vi "Autonomous Path Planner.vi"() -> ()   [LabVIEW 2016]
uses:
  <vilib>/Utility/miscctls.llb/LVCursorListTypeDef.ctl
  <vilib>/Analysis/1siggen.llb/Ramp Pattern by Samples.vi
  Common Code/Utilities/Change Detect String.vi
  <vilib>/Analysis/NI_AALBase.lvlib
  <vilib>/Analysis/NI_AALPro.lvlib
panel:
  in  "Field Lines":T1(array[cluster])=[{"X"=-326.0, "Y"=122.875, "X 2"=-322.0, "Y 2"=122.875}, {"X"=-326.0, "Y"=121.125, "X 2"=-322.0, "Y 2"=121.125}, {"X"=-326.0, "Y"=52.125, "X 2"=-322.0, "Y 2"=52.125}, {"X"=-326.0, "Y"=50.375, "X 2"=-322.0, "Y 2"=50.375}, {"X"=-326.0, "Y"=20.375, "X 2"=-322.0, "Y 2"=20.375}, {"X"=-326.0, "Y"=18.625, "X 2"=-322.0, "Y 2"=18.625}, {"X"=-326.0, "Y"=-50.375, "X 2"=-322.0, "Y 2"=-50.375}, {"X"=-326.0, "Y"=-52.125, "X 2"=-322.0, "Y 2"=-52.125}, {"X"=-326.0, "Y"=-121.125, "X 2"=-322.0, "Y 2"=-121.125}, {"X"=-326.0, "Y"=-122.875, "X 2"=-322.0, "Y 2"=-122.875}, {"X"=0.0, "Y"=0.0, "X 2"=0.0, "Y 2"=0.0}, {"X"=-211.7, "Y"=-20.5, "X 2"=-211.7, "Y 2"=20.5}, {"X"=-140.7, "Y"=-20.5, "X 2"=-140.7, "Y 2"=20.5}, {"X"=-176.2, "Y"=41.0, "X 2"=-211.7, "Y 2"=20.5}, {"X"=-176.2, "Y"=41.0, "X 2"=-140.7, "Y 2"=20.5}, {"X"=-176.2, "Y"=-41.0, "X 2"=-211.7, "Y 2"=-20.5}, {"X"=-176.2, "Y"=-41.0, "X 2"=-140.7, "Y 2"=-20.4}, {"X"=-326.0, "Y"=-126.0, "X 2"=-290.0, "Y 2"=-162.0}, {"X"=-326.0, "Y"=126.0, "X 2"=-254.0, "Y 2"=162.0}, {"X"=-247.5, "Y"=-162.0, "X 2"=-247.5, "Y 2"=-158.0}, {"X"=-221.3, "Y"=-162.0, "X 2"=-221.3, "Y 2"=-158.0}, {"X"=-191.3, "Y"=-162.0, "X 2"=-191.3, "Y 2"=-158.0}, {"X"=-165.1, "Y"=-162.0, "X 2"=-165.1, "Y 2"=-158.0}, {"X"=-41.2, "Y"=-162.0, "X 2"=-41.2, "Y 2"=-158.0}, {"X"=-15.0, "Y"=-162.0, "X 2"=-15.0, "Y 2"=-158.0}, {"X"=-160.5, "Y"=162.0, "X 2"=-160.5, "Y 2"=158.0}, {"X"=-134.3, "Y"=162.0, "X 2"=-134.3, "Y 2"=158.0}, {"X"=-104.3, "Y"=162.0, "X 2"=-104.3, "Y 2"=158.0}, {"X"=-78.1, "Y"=162.0, "X 2"=-78.1, "Y 2"=158.0}, {"X"=-193.95, "Y"=-30.75, "X 2"=-199.2, "Y 2"=-39.84}, {"X"=-193.95, "Y"=30.75, "X 2"=-199.2, "Y 2"=39.84}, {"X"=-211.7, "Y"=0.0, "X 2"=-222.2, "Y 2"=0.0}, {"X"=-211.7, "Y"=-20.5, "X 2"=-233.13, "Y 2"=-32.88}, {"X"=-211.7, "Y"=20.5, "X 2"=-233.13, "Y 2"=32.88}, {"X"=326.0, "Y"=122.875, "X 2"=322.0, "Y 2"=122.875}, {"X"=326.0, "Y"=121.125, "X 2"=322.0, "Y 2"=121.125}, {"X"=326.0, "Y"=52.125, "X 2"=322.0, "Y 2"=52.125}, {"X"=326.0, "Y"=50.375, "X 2"=322.0, "Y 2"=50.375}, {"X"=326.0, "Y"=20.375, "X 2"=322.0, "Y 2"=20.375}, {"X"=326.0, "Y"=18.625, "X 2"=322.0, "Y 2"=18.625}, {"X"=326.0, "Y"=-50.375, "X 2"=322.0, "Y 2"=-50.375}, {"X"=326.0, "Y"=-52.125, "X 2"=322.0, "Y 2"=-52.125}, {"X"=326.0, "Y"=-121.125, "X 2"=322.0, "Y 2"=-121.125}, {"X"=326.0, "Y"=-122.875, "X 2"=322.0, "Y 2"=-122.875}, {"X"=0.0, "Y"=0.0, "X 2"=0.0, "Y 2"=0.0}, {"X"=211.7, "Y"=-20.5, "X 2"=211.7, "Y 2"=20.5}, {"X"=140.7, "Y"=-20.5, "X 2"=140.7, "Y 2"=20.5}, {"X"=176.2, "Y"=41.0, "X 2"=211.7, "Y 2"=20.5}, {"X"=176.2, "Y"=41.0, "X 2"=140.7, "Y 2"=20.5}, {"X"=176.2, "Y"=-41.0, "X 2"=211.7, "Y 2"=-20.5}, {"X"=176.2, "Y"=-41.0, "X 2"=140.7, "Y 2"=-20.4}, {"X"=326.0, "Y"=-126.0, "X 2"=290.0, "Y 2"=-162.0}, {"X"=326.0, "Y"=126.0, "X 2"=254.0, "Y 2"=162.0}, {"X"=247.5, "Y"=-162.0, "X 2"=247.5, "Y 2"=-158.0}, {"X"=221.3, "Y"=-162.0, "X 2"=221.3, "Y 2"=-158.0}, {"X"=191.3, "Y"=-162.0, "X 2"=191.3, "Y 2"=-158.0}, {"X"=165.1, "Y"=-162.0, "X 2"=165.1, "Y 2"=-158.0}, {"X"=41.2, "Y"=-162.0, "X 2"=41.2, "Y 2"=-158.0}, {"X"=15.0, "Y"=-162.0, "X 2"=15.0, "Y 2"=-158.0}, {"X"=160.5, "Y"=162.0, "X 2"=160.5, "Y 2"=158.0}, {"X"=134.3, "Y"=162.0, "X 2"=134.3, "Y 2"=158.0}, {"X"=104.3, "Y"=162.0, "X 2"=104.3, "Y 2"=158.0}, {"X"=78.1, "Y"=162.0, "X 2"=78.1, "Y 2"=158.0}, {"X"=193.95, "Y"=-30.75, "X 2"=199.2, "Y 2"=-39.84}, {"X"=193.95, "Y"=30.75, "X 2"=199.2, "Y 2"=39.84}, {"X"=211.7, "Y"=0.0, "X 2"=222.2, "Y 2"=0.0}, {"X"=211.7, "Y"=-20.5, "X 2"=233.13, "Y 2"=-32.88}, {"X"=211.7, "Y"=20.5, "X 2"=233.13, "Y 2"=32.88}, {"X"=-232.7, "Y"=162.0, "X 2"=-232.7, "Y 2"=-162.0}, {"X"=232.7, "Y"=162.0, "X 2"=232.7, "Y 2"=-162.0}, {"X"=-140.7, "Y"=162.0, "X 2"=-140.7, "Y 2"=-162.0}, {"X"=140.7, "Y"=162.0, "X 2"=140.7, "Y 2"=-162.0}]
  in  "stop":bool
  in  "Graph Tab Control":T2(tab)
  in  "Node Coordinates":cluster{"x":dbl, "y":dbl, "node name":string}[](array[cluster])
  out "Field":T3(graph)
  in  "Zero Direction":bool
  in  "Path Time (sec)":dbl=15.0
  in  "Frequency (ms)":dbl=20.0
  in  "balance parameter":dbl=0.001 step=0.0001
  in  "Robot Width":dbl=36.0 format="%#_13g"
  in  "Auto Balance Param?":bool=TRUE
  in  "Robot Length":dbl=33.0 format="%#_13g"
  in  "Clear List":bool
  in  "In/s       ft/s":bool
  out "Wheel Velocity":cluster{dbl[], dbl[]}[](graph)
  out "Actual Time":dbl
  out "Average Speed Right":dbl
  out "Average Speed Left":dbl
  out "Node Distance":dbl
  out "Points":dbl
  out "Total Distance Traveled":dbl
  out "Distance":cluster{dbl[], dbl[]}(graph)
  out "Angle":cluster{dbl[], dbl[]}(graph)
  # "If the curves are too sharp, try decreasing the balance parameter or try increasing the frequency."
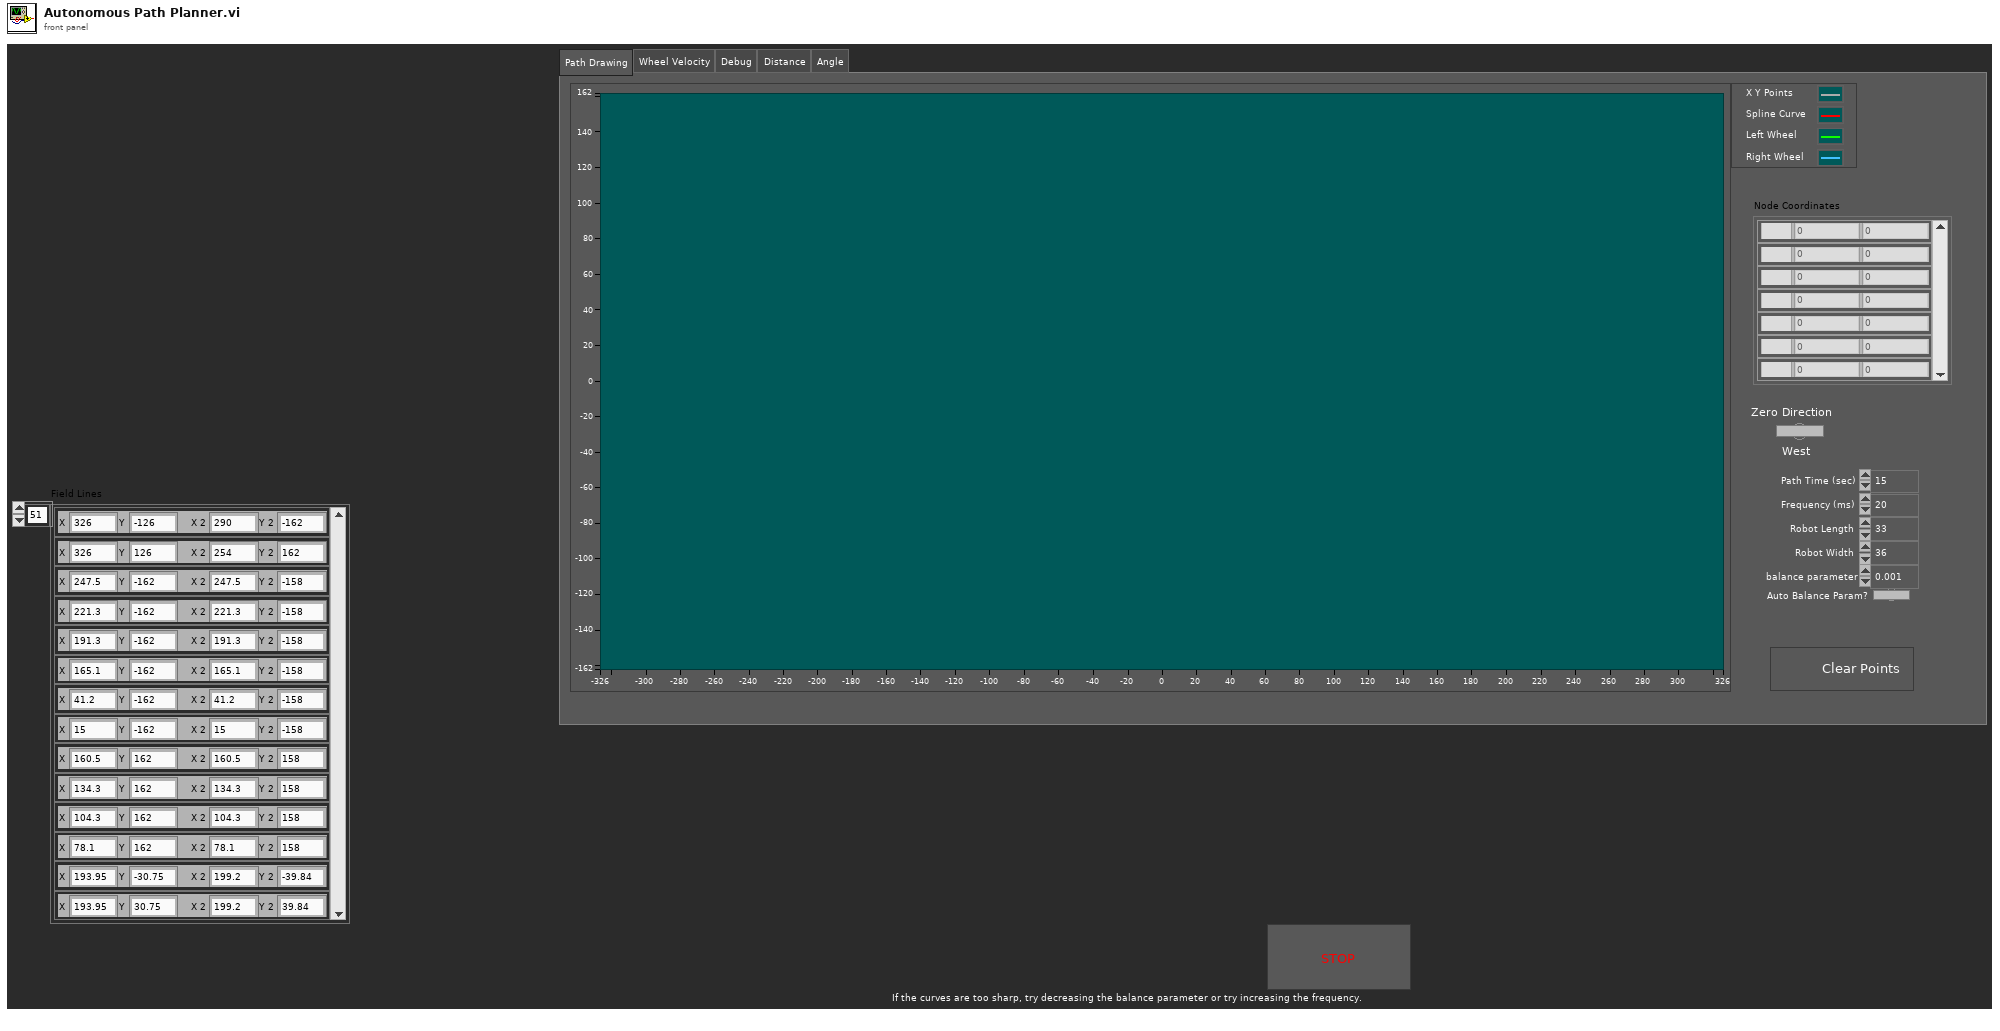
[diagram p1: front panel]
types:
  T1 = cluster{"X":dbl, "Y":dbl, "X 2":dbl, "Y 2":dbl}[]
  T2 = enum32{"Path Drawing", "Wheel Velocity", "Debug", "Distance", "Angle"}
  T3 = cluster{"Best Cubic Spline Fit":dbl[], "Best Cubic Spline Fit":dbl[]}[]
  T4 = cluster{"Name":string, "Color":i32, "Style":i32, "Point Style":i32, "Name Visible":bool, "Allow Drag":bool, "Cursor Mode":u32, "Plot":i32, "Index":i32, "Position":cluster{"X":dbl, "Y":dbl}, "X Scale":u32, "Y Scale":u32, "Watch Plots":i32[], "Watch All Plots":bool, "Plot Area":i32, "Label Offset":cluster{"X":dbl, "Y":dbl}}
  T5 = typedef "LVCursorListTypeDef.ctl" = cluster{"Name":string, "Color":u32, "Style":u8, "Point Style":u8, "Name Visible":bool, "Allow Drag":bool, "Cursor Mode":u32, "Plot":i32, "Index":i32, "Position":cluster{"X":dbl, "Y":dbl}, "X Scale":u32, "Y Scale":u32, "Watch Plots":i32[], "Watch All Plots":bool, "Plot Area":i32, "Label Offset":cluster{"X":dbl, "Y":dbl}}[]
  T6 = typedef "LVPoint32TypeDef.ctl" = cluster{"Horizontal":i32, "Vertical":i32}
  T7 = typedef "LVRectTypeDef.ctl" = cluster{"Left":i16, "Top":i16, "Right":i16, "Bottom":i16}
  T8 = typedef "LVRangeTypeDef.ctl" = cluster{"Minimum":dbl, "Maximum":dbl, "Increment":dbl, "Minor Increment":dbl, "Start":dbl}
  T9 = cluster{"Name":string, "Color":u32, "Style":i32, "Point Style":i32, "Name Visible":bool, "Allow Drag":bool, "Cursor Mode":u32, "Plot":i32, "Index":i32, "Position":cluster{"X":dbl, "Y":dbl}, "X Scale":u32, "Y Scale":u32, "Watch Plots":i32[], "Watch All Plots":bool, "Plot Area":i32, "Label Offset":cluster{"X":dbl, "Y":dbl}}[]
  T10 = typedef "eventvkey.ctl" = enum16{"ASCII", "Enter", "Return", "Shift", "Ctrl", "Alt", "Cmd", "Opt", "Caps", "NumLock", "Clear", "Break", "Up", "Down", "Left", "Right", "Insert", "Delete", "Home", "End", "PageUp", "PageDown", "Escape", "Help", "Pause", "ScrollLock", "F1", "F2", "F3", "F4", "F5", "F6", "F7", "F8", "F9", "F10", "F11", "F12", "F13", "F14", "F15", "F16", "F17", "F18", "F19", "F20", "F21", "F22", "F23", "F24", "Play", "VolumeUp", "VolumeDown", "Mute", "Two Byte Char"}
  T11 = cluster{"Name":string, "Color":u32, "Style":u8, "Point Style":u8, "Name Visible":bool, "Allow Drag":bool, "Cursor Mode":u32, "Plot":i32, "Index":i32, "Position":cluster{"X":dbl, "Y":dbl}, "X Scale":u32, "Y Scale":u32, "Watch Plots":i32[], "Watch All Plots":bool, "Plot Area":i32, "Label Offset":cluster{"X":dbl, "Y":dbl}}
  T12 = cluster{"Best Cubic Spline Fit":dbl[], "Best Cubic Spline Fit":dbl[]}
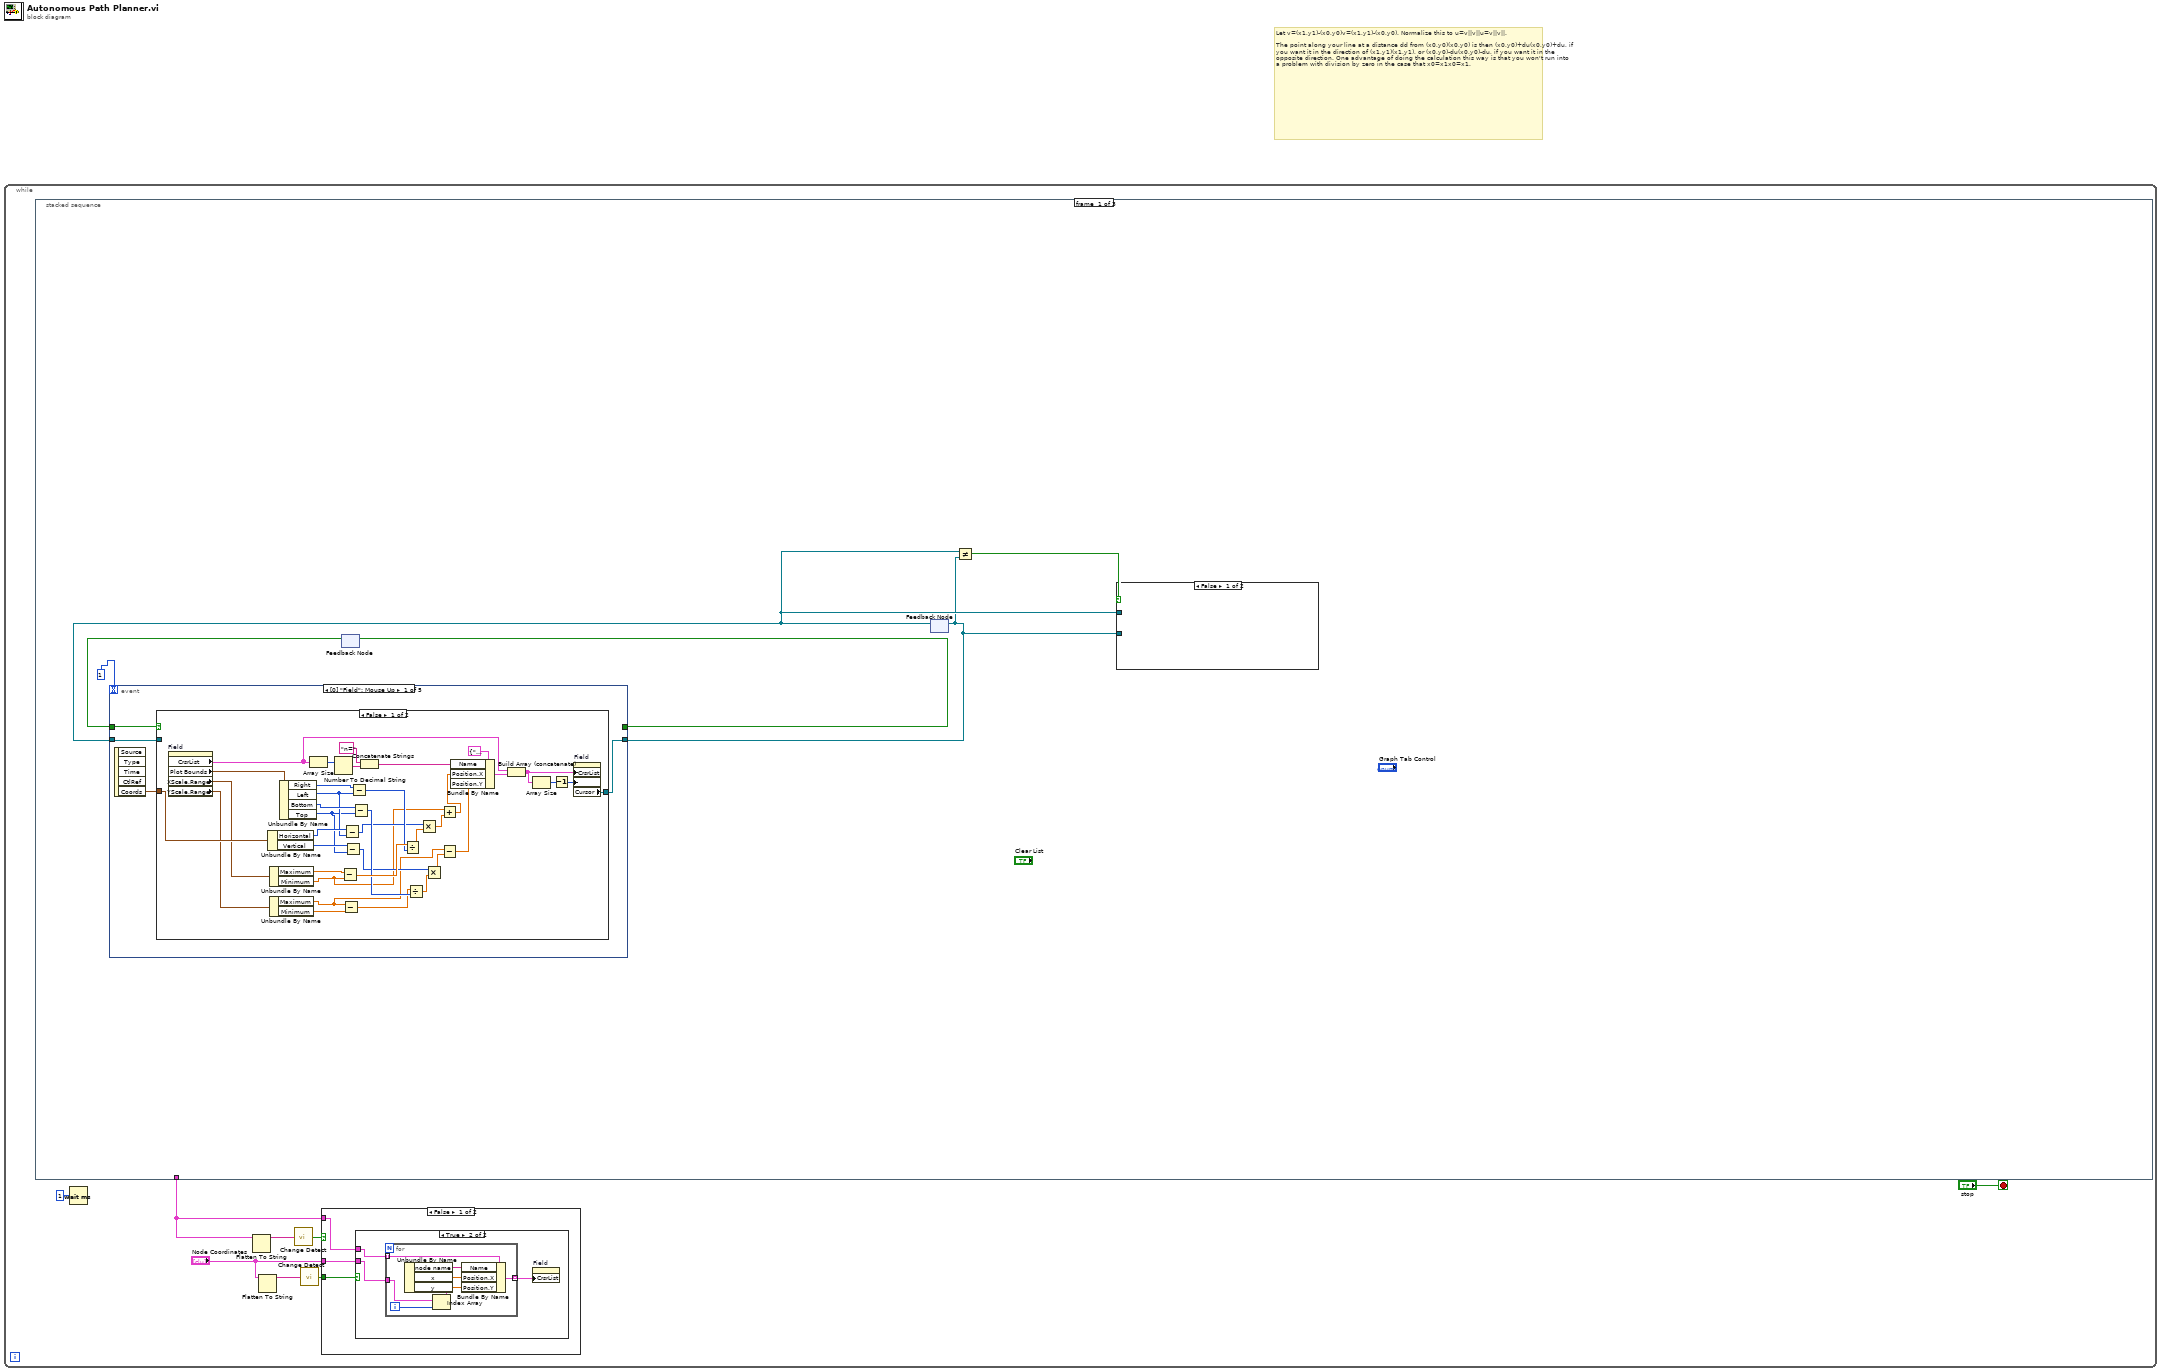
[diagram p0: block diagram]
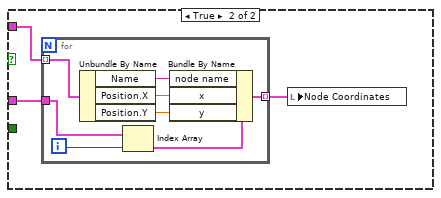
[diagram p3: hidden frame]
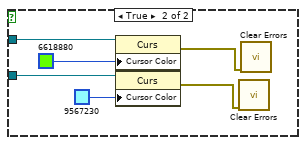
[diagram p4: hidden frame]
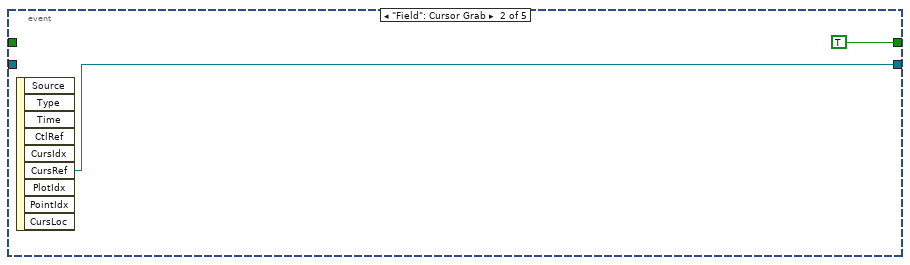
[diagram p6: hidden frame]
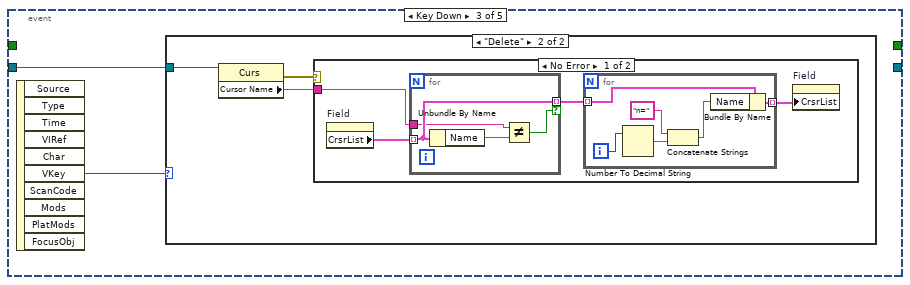
[diagram p7: hidden frame]
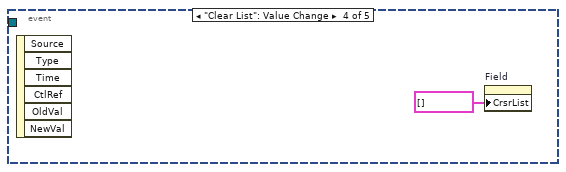
[diagram p10: hidden frame]
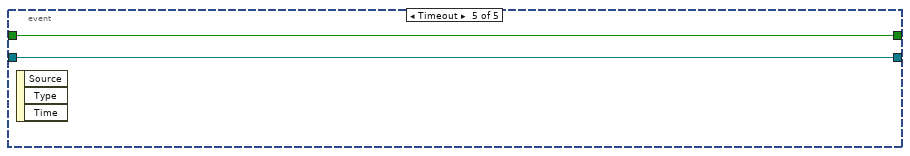
[diagram p11: hidden frame]
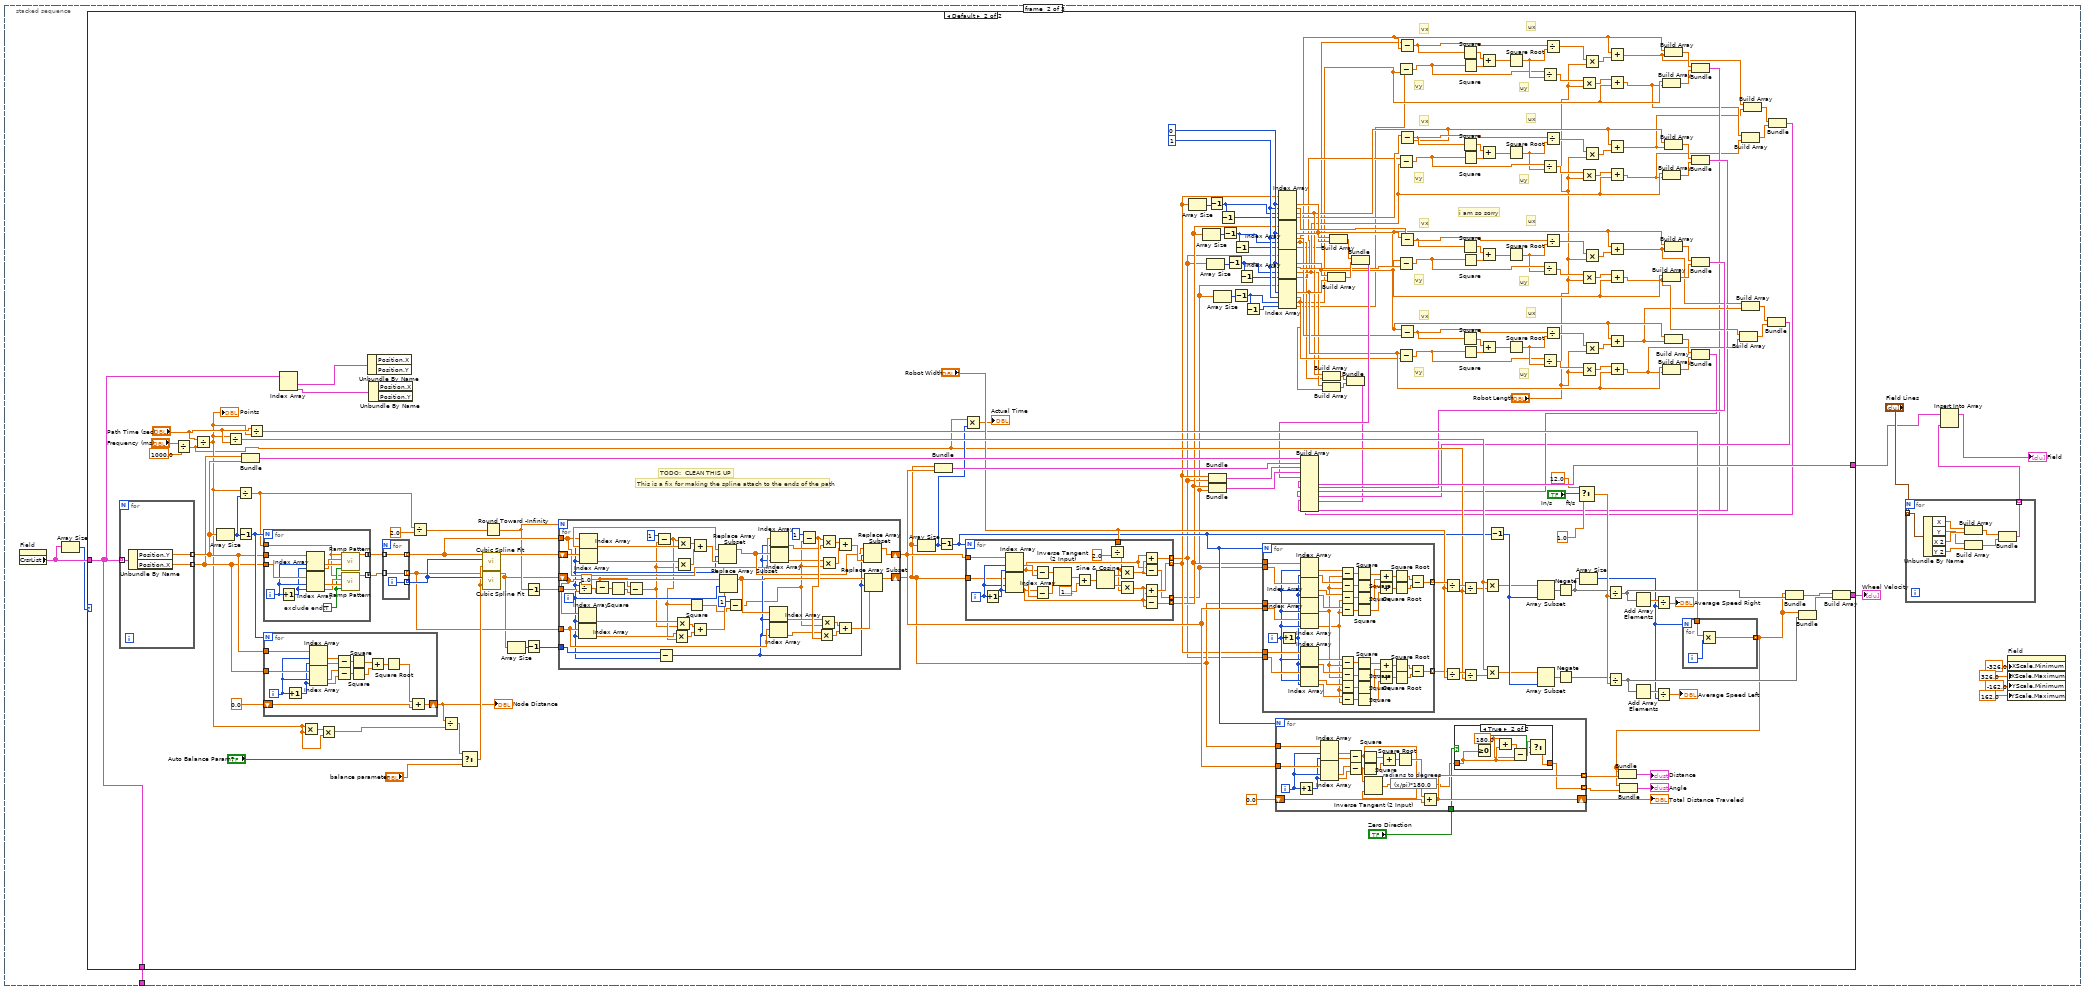
[diagram p12: hidden frame]
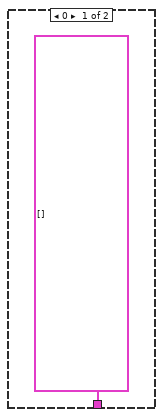
[diagram p13: hidden frame]
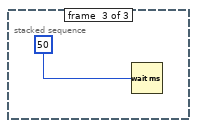
[diagram p15: hidden frame]
diagram:
  # "Let v=(x1,y1)-(x0,y0)v=(x1,y1)-(x0,y0). Normalize this to u=v||v||u=v||v||.\n\nThe point along your line at a distance dd from (x0,y0)(x0,y0) is then (x0,y0)+du(x0,y0)+du, if you want it in the direction of (x1,y1)(x1,y1), or (x0,y0)-du(x0,y0)-du, if you want it in the opposite direction. One advantage of doing the calculation this way is that you won't run into a problem with division by zero in the case that x0=x1x0=x1."
  n1 = while {
    stop <- "stop" stop-if-true
    n2 = stacked-sequence {
      tunnel: [_ w112 _] -> w5
      frame #0 {
        n3 = feedback #1() -> (w38:bool)  [unwired: 1 in]
        n4 = feedback #2() -> (w35:refnum<vi>)  [unwired: 1 in]
        n5 = event shown="[0] \"Field\": Mouse Up" {
          selector: _ -> [_ _ _ _ _]
          dyn-events: _ -> [_ _ _ _ _]
          timeout: 1 -> [_ _ _ _ _]
          tunnel: [_ TRUE _ _ w111] -> w39
          tunnel: w38 -> [w48 _ _ _ w111]
          tunnel: [w47 w88 _ _ w110] -> w34
          tunnel: w35 -> [w46 _ w90 _ w110]
          event "Field": Mouse Up {
            n6 = event-data() -> ("Coords"=w49:T6)  [unwired: 1 in, 4 out]
            n7 = case shown="False" w48 {
              tunnel: w49 -> [w79 _]
              tunnel: [w73 w87] -> w47
              tunnel: w46 -> [_ w87]
              frame False {
                n8 = property on="Field" class="XYGraph (strict)"() -> ("CrsrList"=w80:T5, "Plot Bounds"=w78:T7, "XScale.Range"=w77:T8, "YScale.Range"=w76:T8)  [unwired: 2 in, 2 out]
                n9 = Unbundle By Name(w79) -> ("Horizontal"=w63:i32, "Vertical"=w61:i32)
                n10 = Unbundle By Name(w77) -> ("Maximum"=w69:dbl, "Minimum"=w54:dbl)
                n11 = Unbundle By Name(w76) -> ("Maximum"=w51:dbl, "Minimum"=w68:dbl)
                n12 = Unbundle By Name(w78) -> ("Right"=w71:i16, "Left"=w62:i16, "Bottom"=w70:i16, "Top"=w60:i16)
                n13 = Array Size(array=w80) -> (size(s)=w86:i32)
                n14 = Number To Decimal String(number=w86) -> (decimal integer string=w84:string)  [unwired: 1 in]
                n15 = Subtract(x=w69, y=w54) -> (x-y=w67:dbl)
                n16 = Subtract(x=w51, y=w68) -> (x-y=w64:dbl)
                n17 = Subtract(x=w63, y=w62) -> (x-y=w59:i32)
                n18 = Subtract(x=w61, y=w60) -> (x-y=w57:i32)
                n19 = Subtract(x=w71, y=w62) -> (x-y=w66:i16)
                n20 = Subtract(x=w70, y=w60) -> (x-y=w65:i16)
                n21 = Concatenate Strings("n=" ("string"), w84) -> (w83:string)
                n22 = Divide(x=w67, y=w66) -> (x/y=w58:dbl)
                n23 = Divide(x=w64, y=w65) -> (x/y=w56:dbl)
                n24 = Multiply(x=w59, y=w58) -> (x*y=w55:dbl)
                n25 = Multiply(x=w57, y=w56) -> (x*y=w52:dbl)
                n26 = Add(x=w54, y=w55) -> (x+y=w53:dbl)
                n27 = Subtract(x=w51, y=w52) -> (x-y=w50:dbl)
                n28 = Bundle By Name(cluster=T4 {"Name"="n=0", "Color"=6618880, "Style"=0, "Point Style"=2, "Name Visible"=TRUE, "Allow Drag"=TRUE, "Cursor Mode"=0, "Plot"=0, "Index"=0, "Position"={"X"=0.0, "Y"=0.0}, "X Scale"=0, "Y Scale"=0, "Watch Plots"=[], "Watch All Plots"=FALSE, "Plot Area"=0, "Label Offset"={"X"=0.0, "Y"=14.9626}}, "Name"=w83, "Position.X"=w53, "Position.Y"=w50) -> (w81:T4)
                n29 = Build Array (concatenate)(w80, w81) -> (w75:T9)
                n30 = Array Size(array=w75) -> (size(s)=w74:i32)
                n31 = Decrement(x=w74) -> (x-1=w72:i32)
                n32 = property on="Field" class="XYGraph (strict)"("CrsrList"=w75, "Active Cursor"=w72) -> ("Cursor"=w73:refnum<vi>)  [unwired: 2 in, 2 out]
              }
              frame True {
              }
            }
          }
          event "Field": Cursor Grab {
            n33 = event-data() -> ("CursRef"=w88:refnum<vi>)  [unwired: 1 in, 8 out]
          }
          event Key Down {
            n34 = event-data() -> ("VKey"=w91:T10)  [unwired: 1 in, 9 out]
            n35 = case shown="\"Delete\"" w91 {
              tunnel: w90 -> [_ w94]
              frame Default {
              }
              frame "Delete" {
                n36 = property class="Curs"(reference=w94) -> (error out=w92:errorcluster, "Cursor Name"=w93:string)  [unwired: 1 in, 1 out]
                n37 = case shown="No Error" w92 {
                  tunnel: w93 -> [w97 _]
                  frame No Error {
                    n38 = property on="Field" class="XYGraph (strict)"() -> ("CrsrList"=w98:T5)  [unwired: 2 in, 2 out]
                    n39 = for {
                      tunnel: w98 -> [w108] mode=indexing
                      tunnel: [w108] -> w96 mode=indexing if=w105
                      tunnel: w97 -> [w106]
                      n40 = Unbundle By Name(w108) -> ("Name"=w107:string)
                      n41 = Not Equal?(x=w106, y=w107) -> (x != y?=w105:bool)
                    }
                    n42 = for {
                      tunnel: w96 -> [w101] mode=indexing
                      tunnel: [w99] -> w95 mode=indexing
                      i -> [w103]
                      n43 = Number To Decimal String(number=w103) -> (decimal integer string=w104:string)  [unwired: 1 in]
                      n44 = Concatenate Strings("n=" ("string"), w104) -> (w100:string)
                      n45 = Bundle By Name(cluster=w101, "Name"=w100) -> (w99:T11)
                    }
                    n46 = property on="Field" class="XYGraph (strict)"("CrsrList"=w95) -> ()  [unwired: 2 in, 2 out]
                  }
                  frame Error {
                  }
                }
              }
            }
          }
          event "Clear List": Value Change {
            n47 = event-data() -> ()  [unwired: 1 in, 6 out]
            n48 = property on="Field" class="XYGraph (strict)"("CrsrList"=T5 [] ("Cursor List")) -> ()  [unwired: 2 in, 2 out]
          }
          event Timeout {
            n49 = event-data() -> ()  [unwired: 1 in, 3 out]
          }
        }
        n50 = feedback-in #1(w39) -> ()
        n51 = feedback-in #2(w34) -> ()
        n52 = Not Equal?(x=w35, y=w34) -> (x != y?=w36:bool)
        n53 = case shown="False" w36 {
          tunnel: w35 -> [_ w45]
          tunnel: w34 -> [_ w44]
          frame False {
          }
          frame True {
            n54 = property class="Curs"(reference=w45, "Cursor Color"=u32 6618880) -> (error out=w40:errorcluster)  [unwired: 1 in, 1 out]
            n55 = property class="Curs"(reference=w44, "Cursor Color"=u32 9567230) -> (error out=w41:errorcluster)  [unwired: 1 in, 1 out]
            n56 = call <vilib>:"Clear Errors.vi"("error in (no error)"=w41) -> ()  [unwired: 5 in, 2 out]
            n57 = call <vilib>:"Clear Errors.vi"("error in (no error)"=w40) -> ()  [unwired: 5 in, 2 out]
          }
        }
      }
      frame #1 {
        n58 = property on="Field" class="XYGraph (strict)"() -> ("CrsrList"=w122:T5)  [unwired: 2 in, 2 out]
        n59 = Array Size(array=w122) -> (size(s)=w121:i32)
        n60 = case shown="Default" w121 {
          tunnel: [_ w316] -> w123
          tunnel: [_ w312] -> w118
          tunnel: w122 -> [_ w133]
          tunnel: [T5 [] ("CrsrList") w133] -> w112
          frame 0 {
          }
          frame Default {
            w237 = 1 ("index")
            w239 = 0 ("index")
            # "i am so sorry"
            # "uy"
            # "ux"
            # "vy"
            # "vx"
            # "uy"
            # "ux"
            # "vy"
            # "vx"
            # "uy"
            # "ux"
            # "vy"
            # "vx"
            # "uy"
            # "ux"
            # "vy"
            # "vx"
            # "TODO:  CLEAN THIS UP"
            # "This is a fix for making the spline attach to the ends of the path"
            n61 = for {
              tunnel: w133 -> [w414] mode=indexing
              tunnel: [w413] -> w296 mode=indexing
              tunnel: [w412] -> w295 mode=indexing
              n62 = Unbundle By Name(w414) -> ("Position.Y"=w413:dbl, "Position.X"=w412:dbl)
            }
            n63 = Divide(x="Frequency (ms)", y=1000.0) -> (x/y=w245:dbl)
            n64 = Divide(x="Path Time (sec)", y=w245) -> (x/y=w257:dbl)
            "Points" <- w257
            n65 = Array Size(array=w296) -> (size(s)=w301:i32)
            n66 = Divide(x=w257, y="Path Time (sec)") -> (x/y=w289:dbl)
            n67 = Divide(x=w257, y=w301) -> (x/y=w270:dbl)
            n68 = Decrement(x=w301) -> (x-1=w297:i32)
            n69 = Bundle(w295, w296) -> (w321:cluster{dbl[], dbl[]})  [unwired: 1 out]
            n70 = Divide(x="Path Time (sec)", y=w257) -> (x/y=w256:dbl)
            n71 = for {
              N: w297 -> [_]
              tunnel: w296 -> [w497]
              tunnel: w295 -> [w496]
              tunnel: [w488] -> w311 mode=concatenating
              tunnel: [w487] -> w310 mode=concatenating
              tunnel: w270 -> [w486]
              i -> [w495]
              w489 = TRUE  # exclude end?
              n72 = Increment(x=w495) -> (x+1=w494:i32)
              n73 = Index Array(array=w497, index #1=w495, index #2=w494) -> (element #1=w493:dbl, element #2=w492:dbl)
              n74 = Index Array(array=w496, index #1=w495, index #2=w494) -> (element #1=w491:dbl, element #2=w490:dbl)
              n75 = call-poly <vilib>:"Ramp Pattern.vi"("exclude end?"=w489, "start"=w493, "end"=w492, "samples"=w486) -> ("Ramp Pattern"=w488:dbl[])  [unwired: 6 in, 1 out]
              n76 = call-poly <vilib>:"Ramp Pattern.vi"("exclude end?"=w489, "start"=w491, "end"=w490, "samples"=w486) -> ("Ramp Pattern"=w487:dbl[])  [unwired: 6 in, 1 out]
            }
            n77 = for {
              N: w297 -> [_]
              tunnel: w296 -> [w384]
              tunnel: w295 -> [w383]
              shift-right: [w371] -> w293
              shift-left: 0.0 -> [w369]
              i -> [w382]
              n78 = Increment(x=w382) -> (x+1=w381:i32)
              n79 = Index Array(array=w384, index #1=w382, index #2=w381) -> (element #1=w380:dbl, element #2=w379:dbl)
              n80 = Index Array(array=w383, index #1=w382, index #2=w381) -> (element #1=w378:dbl, element #2=w377:dbl)
              n81 = Subtract(x=w380, y=w379) -> (x-y=w376:dbl)
              n82 = Subtract(x=w378, y=w377) -> (x-y=w375:dbl)
              n83 = Square(x=w376) -> (x^2=w374:dbl)
              n84 = Square(x=w375) -> (x^2=w373:dbl)
              n85 = Add(x=w374, y=w373) -> (x+y=w372:dbl)
              n86 = Square Root(x=w372) -> (sqrt(x)=w370:dbl)
              n87 = Add(x=w370, y=w369) -> (x+y=w371:dbl)
            }
            "Node Distance" <- w293
            n88 = Index Array(array=w133) -> (element #1=w244:T11, element #2=w243:T11)  [unwired: 2 in]
            n89 = Multiply(x=w257, y=w257) -> (x*y=w291:dbl)
            n90 = Multiply(x=w291, y=w257) -> (x*y=w272:dbl)
            n91 = Unbundle By Name(w244) -> ()  [unwired: 2 out]
            n92 = Unbundle By Name(w243) -> ()  [unwired: 2 out]
            n93 = for {
              tunnel: w311 -> [w485] mode=indexing
              tunnel: [w485] -> w274 mode=indexing
              tunnel: [w484] -> w319 mode=indexing
              tunnel: w310 -> [w483] mode=indexing
              tunnel: [w483] -> w271 mode=indexing
              i -> [w484]
            }
            n94 = Divide(x=w270, y=2.0) -> (x/y=w269:dbl)
            n95 = Divide(x=w293, y=w272) -> (x/y=w292:dbl)
            n96 = Select(t=w292, s="Auto Balance Param?", f="balance parameter") -> (s? t:f=w298:dbl)
            n97 = call <vilib>:"Cubic Spline Fit.vi"("Y"=w274, "X"=w319, "balance parameter"=w298) -> ("Best Cubic Spline Fit"=w275:dbl[])  [unwired: 11 in, 1 out]
            n98 = call <vilib>:"Cubic Spline Fit.vi"("Y"=w271, "X"=w319, "balance parameter"=w298) -> ("Best Cubic Spline Fit"=w265:dbl[])  [unwired: 11 in, 1 out]
            n99 = Round Toward -Infinity(1:w269) -> (0:w267:dbl)
            n100 = Array Size(array=w265) -> (size(s)=w264:i32)
            n101 = Decrement(x=w267) -> (x-1=w266:dbl)
            n102 = Decrement(x=w264) -> (x-1=w263:i32)
            n103 = for {
              N: w267 -> [_]
              shift-right: [w335] -> w273
              shift-left: w275 -> [w362]
              tunnel: w274 -> [w338]
              shift-right: [w343] -> w242
              shift-left: w265 -> [w357]
              tunnel: w271 -> [w341]
              tunnel: w266 -> [w355]
              tunnel: w263 -> [w337]
              i -> [w336]
              w326 = 1.0 ("x")
              n104 = Divide(x=w336, y=w355) -> (x/y=w329:dbl)
              n105 = Index Array(array=w357, index=w336) -> (element=w361:dbl)
              n106 = Index Array(array=w341, index=w336) -> (element=w360:dbl)
              n107 = Index Array(array=w338, index=w336) -> (element=w366:dbl)
              n108 = Index Array(array=w362, index=w336) -> (element=w368:dbl)
              n109 = Subtract(x=w326, y=w329) -> (x-y=w328:dbl)
              n110 = Square(x=w328) -> (x^2=w327:dbl)
              n111 = Subtract(x=w326, y=w327) -> (x-y=w325:dbl)
              n112 = Subtract(x=1, y=w325) -> (x-y=w333:dbl)
              n113 = Subtract(x=w337, y=w336) -> (x-y=w334:i32)
              n114 = Multiply(x=w360, y=w333) -> (x*y=w359:dbl)
              n115 = Multiply(x=w361, y=w325) -> (x*y=w358:dbl)
              n116 = Multiply(x=w333, y=w366) -> (x*y=w365:dbl)
              n117 = Multiply(x=w368, y=w325) -> (x*y=w364:dbl)
              n118 = Square(x=w333) -> (x^2=w331:dbl)
              n119 = Add(x=w365, y=w364) -> (x+y=w363:dbl)
              n120 = Add(x=w358, y=w359) -> (x+y=w356:dbl)
              n121 = Replace Array Subset(array=w362, new element=w363, index=w336) -> (w342:dbl[])
              n122 = Replace Array Subset(array=w357, new element=w356, index=w336) -> (w344:dbl[])
              n123 = Subtract(x=1, y=w331) -> (x-y=w330:dbl)
              n124 = Index Array(array=w344, index=w334) -> (element=w350:dbl)
              n125 = Index Array(array=w341, index=w334) -> (element=w340:dbl)
              n126 = Index Array(array=w338, index=w334) -> (element=w339:dbl)
              n127 = Index Array(array=w342, index=w334) -> (element=w345:dbl)
              n128 = Subtract(x=1, y=w330) -> (x-y=w351:dbl)
              n129 = Multiply(x=w340, y=w351) -> (x*y=w352:dbl)
              n130 = Multiply(x=w350, y=w330) -> (x*y=w353:dbl)
              n131 = Multiply(x=w351, y=w339) -> (x*y=w347:dbl)
              n132 = Multiply(x=w345, y=w330) -> (x*y=w348:dbl)
              n133 = Add(x=w347, y=w348) -> (x+y=w349:dbl)
              n134 = Add(x=w353, y=w352) -> (x+y=w354:dbl)
              n135 = Replace Array Subset(array=w342, new element=w349, index=w334) -> (w335:dbl[])
              n136 = Replace Array Subset(array=w344, new element=w354, index=w334) -> (w343:dbl[])
            }
            n137 = Array Size(array=w242) -> (size(s)=w246:i32)
            n138 = Bundle("Best Cubic Spline Fit"=w242, "Best Cubic Spline Fit"=w273) -> (w320:T12)  [unwired: 1 out]
            n139 = Decrement(x=w246) -> (x-1=w254:i32)
            n140 = Multiply(x=w245, y=w246) -> (x*y=→"Actual Time":dbl)
            n141 = for {
              N: w254 -> [_]
              tunnel: w273 -> [w482]
              tunnel: [w473] -> w195 mode=indexing
              tunnel: [w472] -> w188 mode=indexing
              tunnel: [w469] -> w187 mode=indexing
              tunnel: [w468] -> w186 mode=indexing
              tunnel: "Robot Width" -> [w466]
              tunnel: w242 -> [w465]
              i -> [w476]
              n142 = Increment(x=w476) -> (x+1=w477:i32)
              n143 = Index Array(array=w482, index #1=w476, index #2=w477) -> (element #1=w481:dbl, element #2=w470:dbl)
              n144 = Index Array(array=w465, index #1=w476, index #2=w477) -> (element #1=w480:dbl, element #2=w474:dbl)
              n145 = Subtract(x=w470, y=w481) -> (x-y=w464:dbl)
              n146 = Subtract(x=w474, y=w480) -> (x-y=w463:dbl)
              n147 = Inverse Tangent (2 Input)(1:w463, 2:w464) -> (0:w479:dbl)
              n148 = Add(x=w479, y=1.5707963267948966) -> (x+y=w467:dbl)
              n149 = Sine & Cosine(0:w467) -> (1:w461:dbl, 2:w462:dbl)
              n150 = Divide(x=w466, y=2.0) -> (x/y=w460:dbl)
              n151 = Multiply(x=w460, y=w461) -> (x*y=w471:dbl)
              n152 = Multiply(x=w462, y=w460) -> (x*y=w475:dbl)
              n153 = Add(x=w470, y=w471) -> (x+y=w469:dbl)
              n154 = Subtract(x=w470, y=w471) -> (x-y=w468:dbl)
              n155 = Add(x=w475, y=w474) -> (x+y=w473:dbl)
              n156 = Subtract(x=w474, y=w475) -> (x-y=w472:dbl)
            }
            n157 = Array Size(array=w195) -> (size(s)=w194:i32)
            n158 = Array Size(array=w188) -> (size(s)=w191:i32)
            n159 = Array Size(array=w187) -> (size(s)=w190:i32)
            n160 = Decrement(x=w194) -> (x-1=w192:i32)
            n161 = Bundle(w195, w187) -> (w318:cluster{dbl[], dbl[]})  [unwired: 1 out]
            n162 = Bundle(w188, w186) -> (w317:cluster{dbl[], dbl[]})  [unwired: 1 out]
            n163 = Array Size(array=w186) -> (size(s)=w189:i32)
            n164 = Decrement(x=w192) -> (x-1=w193:i32)
            n165 = Decrement(x=w191) -> (x-1=w181:i32)
            n166 = Decrement(x=w190) -> (x-1=w183:i32)
            n167 = Decrement(x=w189) -> (x-1=w184:i32)
            n168 = Decrement(x=w181) -> (x-1=w180:i32)
            n169 = Decrement(x=w183) -> (x-1=w182:i32)
            n170 = Decrement(x=w184) -> (x-1=w185:i32)
            n171 = for {
              N: w254 -> [_]
              tunnel: w186 -> [w457]
              tunnel: w188 -> [w458]
              tunnel: w242 -> [w456]
              tunnel: w273 -> [w455]
              tunnel: [w415] -> w286 mode=indexing
              tunnel: w195 -> [w424]
              tunnel: w187 -> [w423]
              tunnel: [w420] -> w283 mode=indexing
              i -> [w419]
              n172 = Increment(x=w419) -> (x+1=w418:i32)
              n173 = Index Array(array=w458, index #1=w419, index #2=w418) -> (element #1=w446:dbl, element #2=w445:dbl)
              n174 = Index Array(array=w457, index #1=w419, index #2=w418) -> (element #1=w444:dbl, element #2=w443:dbl)
              n175 = Index Array(array=w456, index=w419) -> (element=w422:dbl)
              n176 = Index Array(array=w455, index=w419) -> (element=w421:dbl)
              n177 = Index Array(array=w424, index #1=w419, index #2=w418) -> (element #1=w430:dbl, element #2=w429:dbl)
              n178 = Index Array(array=w423, index #1=w419, index #2=w418) -> (element #1=w428:dbl, element #2=w427:dbl)
              n179 = Subtract(x=w446, y=w422) -> (x-y=w454:dbl)
              n180 = Subtract(x=w445, y=w422) -> (x-y=w453:dbl)
              n181 = Subtract(x=w444, y=w421) -> (x-y=w452:dbl)
              n182 = Subtract(x=w443, y=w421) -> (x-y=w451:dbl)
              n183 = Subtract(x=w430, y=w422) -> (x-y=w440:dbl)
              n184 = Subtract(x=w429, y=w422) -> (x-y=w439:dbl)
              n185 = Subtract(x=w428, y=w421) -> (x-y=w438:dbl)
              n186 = Subtract(x=w427, y=w421) -> (x-y=w437:dbl)
              n187 = Square(x=w454) -> (x^2=w450:dbl)
              n188 = Square(x=w453) -> (x^2=w449:dbl)
              n189 = Square(x=w452) -> (x^2=w442:dbl)
              n190 = Square(x=w451) -> (x^2=w441:dbl)
              n191 = Square(x=w440) -> (x^2=w436:dbl)
              n192 = Square(x=w439) -> (x^2=w435:dbl)
              n193 = Square(x=w438) -> (x^2=w426:dbl)
              n194 = Square(x=w437) -> (x^2=w425:dbl)
              n195 = Add(x=w450, y=w442) -> (x+y=w448:dbl)
              n196 = Add(x=w449, y=w441) -> (x+y=w447:dbl)
              n197 = Add(x=w436, y=w426) -> (x+y=w434:dbl)
              n198 = Add(x=w435, y=w425) -> (x+y=w433:dbl)
              n199 = Square Root(x=w448) -> (sqrt(x)=w416:dbl)
              n200 = Square Root(x=w447) -> (sqrt(x)=w417:dbl)
              n201 = Square Root(x=w434) -> (sqrt(x)=w432:dbl)
              n202 = Square Root(x=w433) -> (sqrt(x)=w431:dbl)
              n203 = Subtract(x=w416, y=w417) -> (x-y=w415:dbl)
              n204 = Subtract(x=w432, y=w431) -> (x-y=w420:dbl)
            }
            n205 = for {
              N: w254 -> [_]
              tunnel: w242 -> [w404]
              tunnel: w273 -> [w403]
              shift-right: [w391] -> w308
              shift-left: 0.0 -> [w392]
              tunnel: [w391] -> w252 mode=indexing
              tunnel: [w385] -> w250 mode=indexing
              tunnel: "Zero Direction" -> [w387]
              i -> [w402]
              n206 = Increment(x=w402) -> (x+1=w401:i32)
              n207 = Index Array(array=w404, index #1=w402, index #2=w401) -> (element #1=w400:dbl, element #2=w399:dbl)
              n208 = Index Array(array=w403, index #1=w402, index #2=w401) -> (element #1=w398:dbl, element #2=w397:dbl)
              n209 = Subtract(x=w400, y=w399) -> (x-y=w389:dbl)
              n210 = Subtract(x=w398, y=w397) -> (x-y=w390:dbl)
              n211 = Square(x=w389) -> (x^2=w396:dbl)
              n212 = Square(x=w390) -> (x^2=w395:dbl)
              n213 = Inverse Tangent (2 Input)(1:w389, 2:w390) -> (0:w388:dbl)
              n214 = Add(x=w396, y=w395) -> (x+y=w394:dbl)
              n215 = expression code="(x/pi)*180.0" "radians to degrees"(w388) -> (w386:dbl)
              n216 = Square Root(x=w394) -> (sqrt(x)=w393:dbl)
              n217 = Add(x=w393, y=w392) -> (x+y=w391:dbl)
              n218 = case shown="True" w387 {
                tunnel: w386 -> [w405 w411]
                tunnel: [w405 w406] -> w385
                frame False {
                }
                frame True {
                  w410 = 180.0 ("x")
                  n219 = Greater Or Equal To 0?(x=w411) -> (x >= 0?=w407:bool)
                  n220 = Add(x=w410, y=w411) -> (x+y=w408:dbl)
                  n221 = Subtract(x=w411, y=w410) -> (x-y=w409:dbl)
                  n222 = Select(t=w409, s=w407, f=w408) -> (s? t:f=w406:dbl)
                }
              }
            }
            "Total Distance Traveled" <- w308
            n223 = Index Array(array=w195, index #1=w239, index #2=w237, index #3=w192, index #4=w193) -> (element #1=w224:dbl, element #2=w236:dbl, element #3=w152:dbl, element #4=w151:dbl)
            n224 = Index Array(array=w188, index #1=w239, index #2=w237, index #3=w181, index #4=w180) -> (element #1=w207:dbl, element #2=w203:dbl, element #3=w148:dbl, element #4=w147:dbl)
            n225 = Index Array(array=w187, index #1=w239, index #2=w237, index #3=w183, index #4=w182) -> (element #1=w223:dbl, element #2=w235:dbl, element #3=w150:dbl, element #4=w149:dbl)
            n226 = Index Array(array=w186, index #1=w239, index #2=w237, index #3=w184, index #4=w185) -> (element #1=w206:dbl, element #2=w205:dbl, element #3=w146:dbl, element #4=w145:dbl)
            n227 = Build Array(w152, w148) -> (w179:dbl[])
            n228 = Build Array(w150, w146) -> (w178:dbl[])
            n229 = Build Array(w223, w206) -> (w241:dbl[])
            n230 = Build Array(w224, w207) -> (w240:dbl[])
            n231 = Bundle(w179, w178) -> (w177:cluster{dbl[], dbl[]})  [unwired: 1 in]
            n232 = Bundle(w240, w241) -> (w238:cluster{dbl[], dbl[]})  [unwired: 1 in]
            n233 = Subtract(x=w145, y=w146) -> (x-y=w157:dbl)
            n234 = Subtract(x=w149, y=w150) -> (x-y=w172:dbl)
            n235 = Subtract(x=w223, y=w235) -> (x-y=w230:dbl)
            n236 = Subtract(x=w206, y=w205) -> (x-y=w212:dbl)
            n237 = Subtract(x=w147, y=w148) -> (x-y=w156:dbl)
            n238 = Subtract(x=w151, y=w152) -> (x-y=w173:dbl)
            n239 = Subtract(x=w224, y=w236) -> (x-y=w231:dbl)
            n240 = Subtract(x=w207, y=w203) -> (x-y=w211:dbl)
            n241 = Divide(x=w286, y="Robot Width") -> (x/y=w285:dbl[])
            n242 = Divide(x=w283, y="Robot Width") -> (x/y=w282:dbl[])
            n243 = Square(x=w156) -> (x^2=w154:dbl)
            n244 = Square(x=w173) -> (x^2=w175:dbl)
            n245 = Square(x=w231) -> (x^2=w233:dbl)
            n246 = Square(x=w211) -> (x^2=w209:dbl)
            n247 = Square(x=w157) -> (x^2=w153:dbl)
            n248 = Square(x=w172) -> (x^2=w176:dbl)
            n249 = Square(x=w230) -> (x^2=w234:dbl)
            n250 = Square(x=w212) -> (x^2=w208:dbl)
            n251 = Divide(x=w285, y=w245) -> (x/y=w287:dbl[])
            n252 = Divide(x=w282, y=w245) -> (x/y=w281:dbl[])
            n253 = Add(x=w154, y=w153) -> (x+y=w155:dbl)
            n254 = Add(x=w175, y=w176) -> (x+y=w174:dbl)
            n255 = Add(x=w233, y=w234) -> (x+y=w232:dbl)
            n256 = Add(x=w209, y=w208) -> (x+y=w210:dbl)
            n257 = Multiply(x=w289, y=w287) -> (x*y=w290:dbl[])
            n258 = Multiply(x=w289, y=w281) -> (x*y=w288:dbl[])
            n259 = Decrement(x=w254) -> (x-1=w314:i32)
            n260 = Square Root(x=w155) -> (sqrt(x)=w158:dbl)
            n261 = Square Root(x=w174) -> (sqrt(x)=w171:dbl)
            n262 = Square Root(x=w232) -> (sqrt(x)=w229:dbl)
            n263 = Square Root(x=w210) -> (sqrt(x)=w213:dbl)
            n264 = Array Subset(array=w290, length=w314) -> (w315:dbl[])  [unwired: 1 in]
            n265 = Array Subset(array=w288, length=w314) -> (w313:dbl[])  [unwired: 1 in]
            n266 = Divide(x=w157, y=w158) -> (x/y=w160:dbl)
            n267 = Divide(x=w172, y=w171) -> (x/y=w169:dbl)
            n268 = Divide(x=w230, y=w229) -> (x/y=w227:dbl)
            n269 = Divide(x=w212, y=w213) -> (x/y=w215:dbl)
            n270 = Divide(x=w156, y=w158) -> (x/y=w159:dbl)
            n271 = Divide(x=w173, y=w171) -> (x/y=w170:dbl)
            n272 = Divide(x=w231, y=w229) -> (x/y=w228:dbl)
            n273 = Divide(x=w211, y=w213) -> (x/y=w214:dbl)
            n274 = Negate(x=w315) -> (-x=w255:dbl[])
            n275 = Negate(x=w313) -> (-x=w278:dbl[])
            n276 = Select(t=12.0, s="In/s       ft/s", f=1.0) -> (s? t:f=w304:dbl)
            n277 = Array Size(array=w255) -> (size(s)=w253:i32)
            n278 = Multiply(x=w160, y="Robot Length") -> (x*y=w162:dbl)
            n279 = Multiply(x=w169, y="Robot Length") -> (x*y=w167:dbl)
            n280 = Multiply(x=w227, y="Robot Length") -> (x*y=w225:dbl)
            n281 = Multiply(x=w215, y="Robot Length") -> (x*y=w217:dbl)
            n282 = Multiply(x=w159, y="Robot Length") -> (x*y=w161:dbl)
            n283 = Multiply(x=w170, y="Robot Length") -> (x*y=w168:dbl)
            n284 = Multiply(x=w228, y="Robot Length") -> (x*y=w226:dbl)
            n285 = Multiply(x=w214, y="Robot Length") -> (x*y=w216:dbl)
            n286 = Divide(x=w255, y=w304) -> (x/y=w261:dbl[])
            n287 = Divide(x=w278, y=w304) -> (x/y=w260:dbl[])
            n288 = Add(x=w148, y=w161) -> (x+y=w138:dbl)
            n289 = Add(x=w162, y=w146) -> (x+y=w137:dbl)
            n290 = Add(x=w152, y=w168) -> (x+y=w136:dbl)
            n291 = Add(x=w167, y=w150) -> (x+y=w135:dbl)
            n292 = Add(x=w224, y=w226) -> (x+y=w202:dbl)
            n293 = Add(x=w225, y=w223) -> (x+y=w201:dbl)
            n294 = Add(x=w207, y=w216) -> (x+y=w200:dbl)
            n295 = Add(x=w217, y=w206) -> (x+y=w199:dbl)
            n296 = Add Array Elements(numeric array=w261) -> (sum=w280:dbl)
            n297 = Add Array Elements(numeric array=w260) -> (sum=w277:dbl)
            n298 = Divide(x=w280, y=w253) -> (x/y=→"Average Speed Right":dbl)
            n299 = Divide(x=w277, y=w253) -> (x/y=→"Average Speed Left":dbl)
            n300 = Build Array(w146, w137) -> (w164:dbl[])
            n301 = Build Array(w150, w135) -> (w165:dbl[])
            n302 = Build Array(w223, w201) -> (w221:dbl[])
            n303 = Build Array(w206, w199) -> (w219:dbl[])
            n304 = Build Array(w148, w138) -> (w163:dbl[])
            n305 = Build Array(w152, w136) -> (w166:dbl[])
            n306 = Build Array(w224, w202) -> (w222:dbl[])
            n307 = Build Array(w207, w200) -> (w218:dbl[])
            n308 = for {
              N: w253 -> [_]
              tunnel: [w323] -> w249 mode=indexing
              tunnel: w256 -> [w322]
              i -> [w324]
              n309 = Multiply(x=w322, y=w324) -> (x*y=w323:dbl)
            }
            n310 = Bundle(w249, w252) -> (→"Distance":cluster{dbl[], dbl[]})  [unwired: 1 out]
            n311 = Bundle(w249, w250) -> (→"Angle":cluster{dbl[], dbl[]})  [unwired: 1 out]
            n312 = Bundle(w163, w164) -> (w142:cluster{dbl[], dbl[]})  [unwired: 1 in]
            n313 = Bundle(w166, w165) -> (w143:cluster{dbl[], dbl[]})  [unwired: 1 in]
            n314 = Bundle(w222, w221) -> (w220:cluster{dbl[], dbl[]})  [unwired: 1 in]
            n315 = Bundle(w218, w219) -> (w204:cluster{dbl[], dbl[]})  [unwired: 1 in]
            n316 = Build Array(w201, w199) -> (w198:dbl[])
            n317 = Build Array(w137, w135) -> (w140:dbl[])
            n318 = Build Array(w202, w200) -> (w197:dbl[])
            n319 = Build Array(w138, w136) -> (w141:dbl[])
            n320 = Bundle(w197, w198) -> (w196:cluster{dbl[], dbl[]})  [unwired: 1 in]
            n321 = Bundle(w141, w140) -> (w139:cluster{dbl[], dbl[]})  [unwired: 1 in]
            n322 = Build Array(w321, w320, w318, w317, w238, w220, w204, w196, w177, w143, w142, w139) -> (w312:T3)
            n323 = Bundle(w249, w261) -> (w262:cluster{dbl[], dbl[]})  [unwired: 1 out]
            n324 = Bundle(w249, w260) -> (w259:cluster{dbl[], dbl[]})  [unwired: 1 out]
            n325 = Build Array(w262, w259) -> (w316:cluster{dbl[], dbl[]}[])
          }
        }
        "Wheel Velocity" <- w123
        n326 = for {
          tunnel: "Field Lines" -> [w131] mode=indexing
          tunnel: [w124] -> w117 mode=indexing
          n327 = Unbundle By Name(w131) -> ("X"=w130:dbl, "Y"=w125:dbl, "X 2"=w126:dbl, "Y 2"=w129:dbl)
          n328 = Build Array(w130, w126) -> (w128:dbl[])
          n329 = Build Array(w125, w129) -> (w127:dbl[])
          n330 = Bundle(w128, w127) -> (w124:cluster{dbl[], dbl[]})  [unwired: 1 in]
        }
        n331 = Insert Into Array(array=w118, new element=w117) -> (→"Field":T3)  [unwired: 1 in]
        n332 = property on="Field" class="XYGraph (strict)"("XScale.Minimum"=-326.0 ("X Scale.Range:Minimum"), "XScale.Maximum"=326.0 ("X Scale.Range:Maximum"), "YScale.Minimum"=-162.0 ("Y Scale.Range:Minimum"), "YScale.Maximum"=162.0 ("Y Scale.Range:Maximum")) -> ()  [unwired: 2 in, 2 out]
      }
      frame #2 {
        n333 = Wait (ms)(milliseconds to wait=u32 50) -> ()  [unwired: 1 out]
      }
    }
    n334 = Wait (ms)(milliseconds to wait=u32 1) -> ()  [unwired: 1 out]
    n335 = Flatten To String(anything=w5) -> (data string=w4:string)  [unwired: 3 in, 2 out]
    n336 = Flatten To String(anything="Node Coordinates") -> (data string=w3:string)  [unwired: 3 in, 2 out]
    n337 = call-poly "Change Detect.vi"("In"=w4) -> ("Changed?"=w6:bool)
    n338 = call-poly "Change Detect.vi"("In"=w3) -> ("Changed?"=w1:bool)
    n339 = case shown="False" w6 {
      tunnel: w5 -> [w10 w24]
      tunnel: "Node Coordinates" -> [w9 w25]
      tunnel: w1 -> [w11 _]
      frame False {
        n340 = case shown="True" w11 {
          tunnel: w10 -> [_ w14]
          tunnel: w9 -> [_ w13]
          frame False {
          }
          frame True {
            n341 = for {
              tunnel: w14 -> [w16] mode=indexing
              tunnel: w13 -> [w18]
              tunnel: [w19] -> w12 mode=indexing
              i -> [w17]
              n342 = Index Array(array=w18, index=w17) -> (element=w15:cluster{"x":dbl, "y":dbl, "node name":string})
              n343 = Unbundle By Name(w15) -> ("node name"=w22:string, "x"=w21:dbl, "y"=w20:dbl)
              n344 = Bundle By Name(cluster=w16, "Name"=w22, "Position.X"=w21, "Position.Y"=w20) -> (w19:T11)
            }
            n345 = property on="Field" class="XYGraph (strict)"("CrsrList"=w12) -> ()  [unwired: 2 in, 2 out]
          }
        }
      }
      frame True {
        n346 = for {
          tunnel: w24 -> [w33] mode=indexing
          tunnel: w25 -> [w28]
          tunnel: [w29] -> w23 mode=indexing
          i -> [w27]
          n347 = Unbundle By Name(w33) -> ("Name"=w32:string, "Position.X"=w31:dbl, "Position.Y"=w30:dbl)
          n348 = Index Array(array=w28, index=w27) -> (element=w26:cluster{"x":dbl, "y":dbl, "node name":string})
          n349 = Bundle By Name(cluster=w26, "node name"=w32, "x"=w31, "y"=w30) -> (w29:cluster{"x":dbl, "y":dbl, "node name":string})
        }
        n350 = local write "Node Coordinates"(w23) -> ()
      }
    }
  }
